vi "Drive.vi"   [LabVIEW 2013]
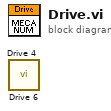
[diagram p0: block diagram]
diagram:
  n1 = call "Drive 6.vi"() -> ()  [unwired: 8 in, 4 out]
  n2 = call "Drive 4.vi"() -> ()  [unwired: 9 in, 3 out]
